vi "Initialize.vi"(8 "error in (no error)":errorcluster) -> (0 "error out":errorcluster, 3 "Mediator out":refnum<class "Mediator.lvclass">)   [LabVIEW 2015, in "Mediator.lvlib" / "Mediator.lvclass"]
doc: "Creates a new Mediator"
uses:
  Mediator.lvclass
  Sequence/Sequence.lvclass
  Controls/Sequence Return Info.ctl
  Mediator.lvclass/Mediator.ctl
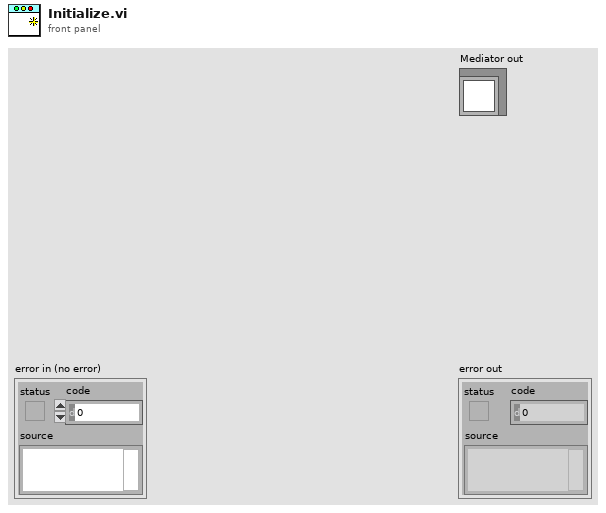
[diagram p1: front panel]
types:
  T1 = typedef "Mediator.lvlib/Sequence.lvclass/Sequence Return Info.ctl" = cluster{"Name":string, "Error Out":errorcluster, "Sequence Parameters out":variant}
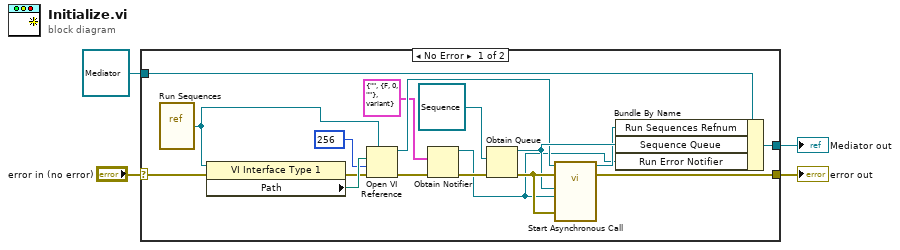
[diagram p0: block diagram]
diagram:
  n1 = case shown="No Error" "error in (no error)" {
    selector: "error in (no error)" -> [w11 w23]
    tunnel: [w18 w23] -> w3
    tunnel: [w19 w22] -> w1
    tunnel: refnum<class "Mediator.lvclass"> refnum ("Mediator in") -> [w20 w22]
    frame No Error {
      n2 = vi-ref "Run Sequences.vi"() -> (w6:refnum<vi>)
      n3 = property class="VI Interface Type 1"(reference=w6, error in=w11) -> (error out=w10:errorcluster, "Path"=w16:path)  [unwired: 1 out]
      n4 = Open VI Reference(type specifier VI Refnum (for type only)=w6, vi path=w16, options=256, error in (no error)=w10) -> (vi reference=w13:refnum<vi>, error out=w9:errorcluster)  [unwired: 2 in]
      n5 = Obtain Notifier(notification data type=T1 {"Name"="", "Error Out"={"status"=FALSE, "code"=0, "source"=""}, "Sequence Parameters out"=variant}, error in (no error)=w9) -> (notifier out=w5:refnum<notifier>, error out=w8:errorcluster)  [unwired: 2 in, 1 out]
      n6 = Obtain Queue(element data type=refnum<class "Sequence.lvclass"> refnum ("SLSC Mediator API.lvlib:Sequence.lvclass"), error in (no error)=w8) -> (queue out=w14:refnum<queue>, error out=w17:errorcluster)  [unwired: 3 in, 1 out]
      n7 = call-by-ref "Start Asynchronous Call"(reference=w13, error in=w17, 8:"error in (no error)"=w17, "Error Notifier in"=w5, "Sequence Queue in"=w14) -> (reference out=w12:refnum<vi>, error out=w18:errorcluster)  [unwired: 8 in, 1 out]
      n8 = Bundle By Name(cluster=w20, "Run Sequences Refnum"=w12, "Sequence Queue"=w14, "Run Error Notifier"=w5) -> (w19:refnum<class "Mediator.lvclass">)
    }
    frame Error {
    }
  }
  "error out" <- w3
  "Mediator out" <- w1
